vi "Add Children.vi"(8 "Error In":errorcluster, 10 "Parent Index":i32, 11 "DFS Data In":T1) -> (0 "Error Out":errorcluster, 3 "DFS Data Out":T1)   [LabVIEW 2022 SP3]
doc: "<add documentation here>"
uses:
  DFS Data (cluster).ctl
  DFS Node (cluster).ctl
  DFS Child Node (cluster).ctl
panel:
  # "Development\nControls or indicators that are useful for development or testing, but which are not outputs of the VI."
  # "Input\nInputs to the VI"
  # "Output\nOutputs of the VI"
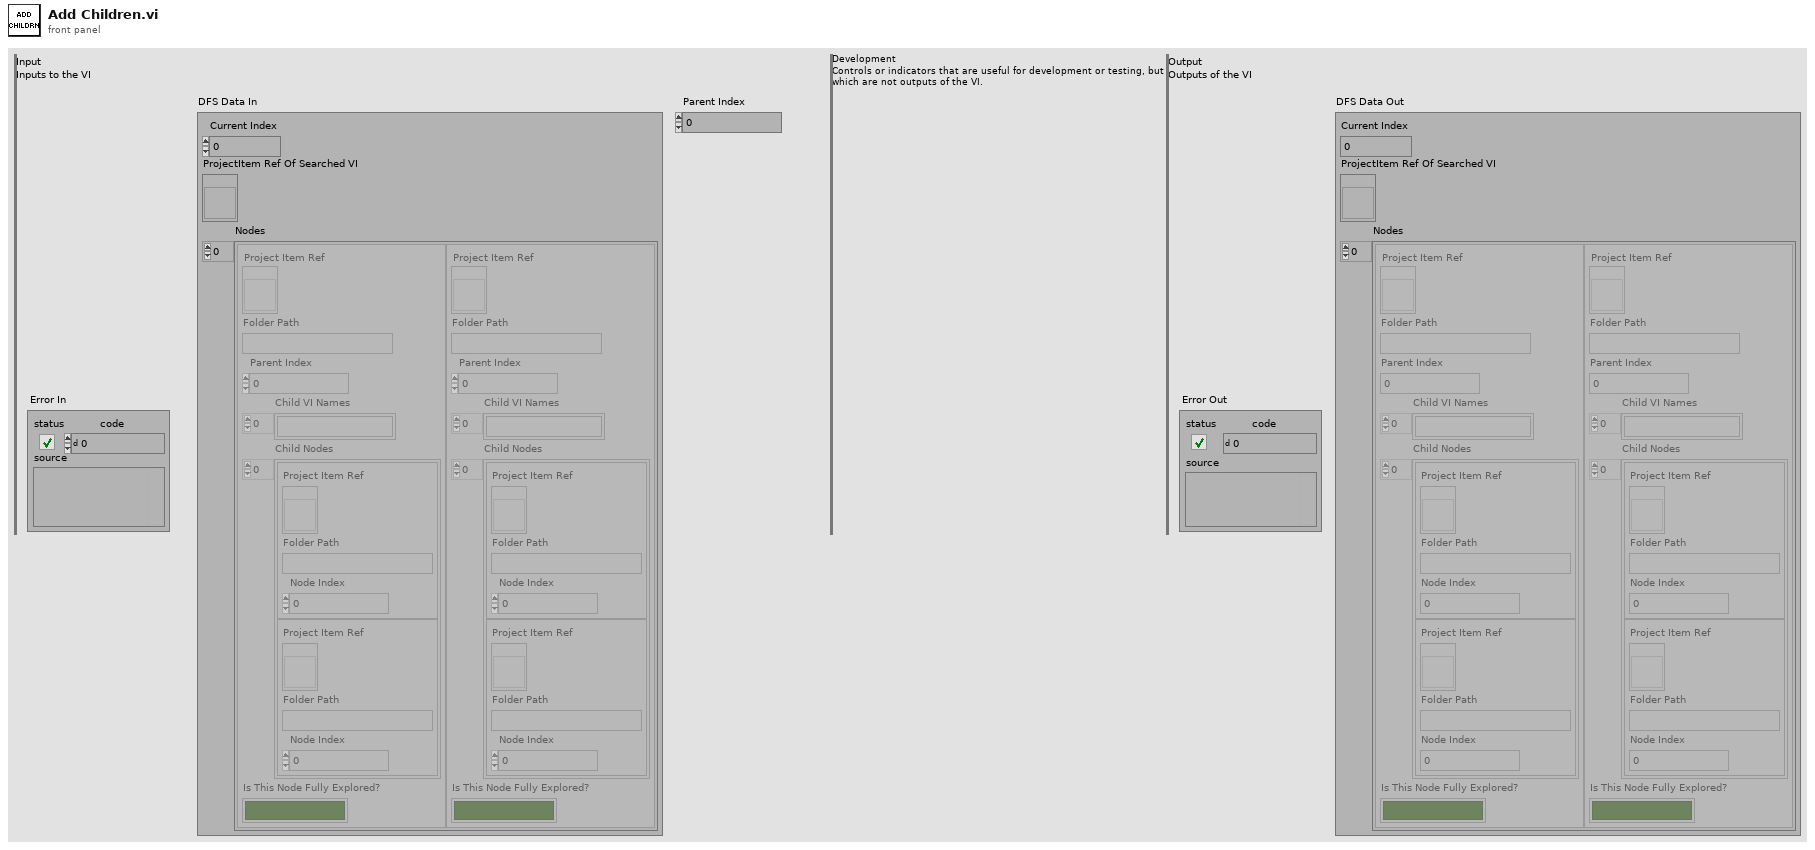
[diagram p1: front panel]
types:
  T1 = typedef "DFS Data (cluster).ctl" = cluster{"Current Index":i32, "ProjectItem Ref Of Searched VI":refnum<vi>, "Nodes":T2[]}
  T2 = typedef "DFS Node (cluster).ctl" = cluster{"Project Item Ref":refnum<vi>, "Folder Path":string, "Parent Index":i32, "Child VI Names":string[], "Child Nodes":T3[], "Is This Node Fully Explored?":bool}
  T3 = typedef "DFS Child Node (cluster).ctl" = cluster{"Project Item Ref":refnum<vi>, "Folder Path":string, "Node Index":i32}
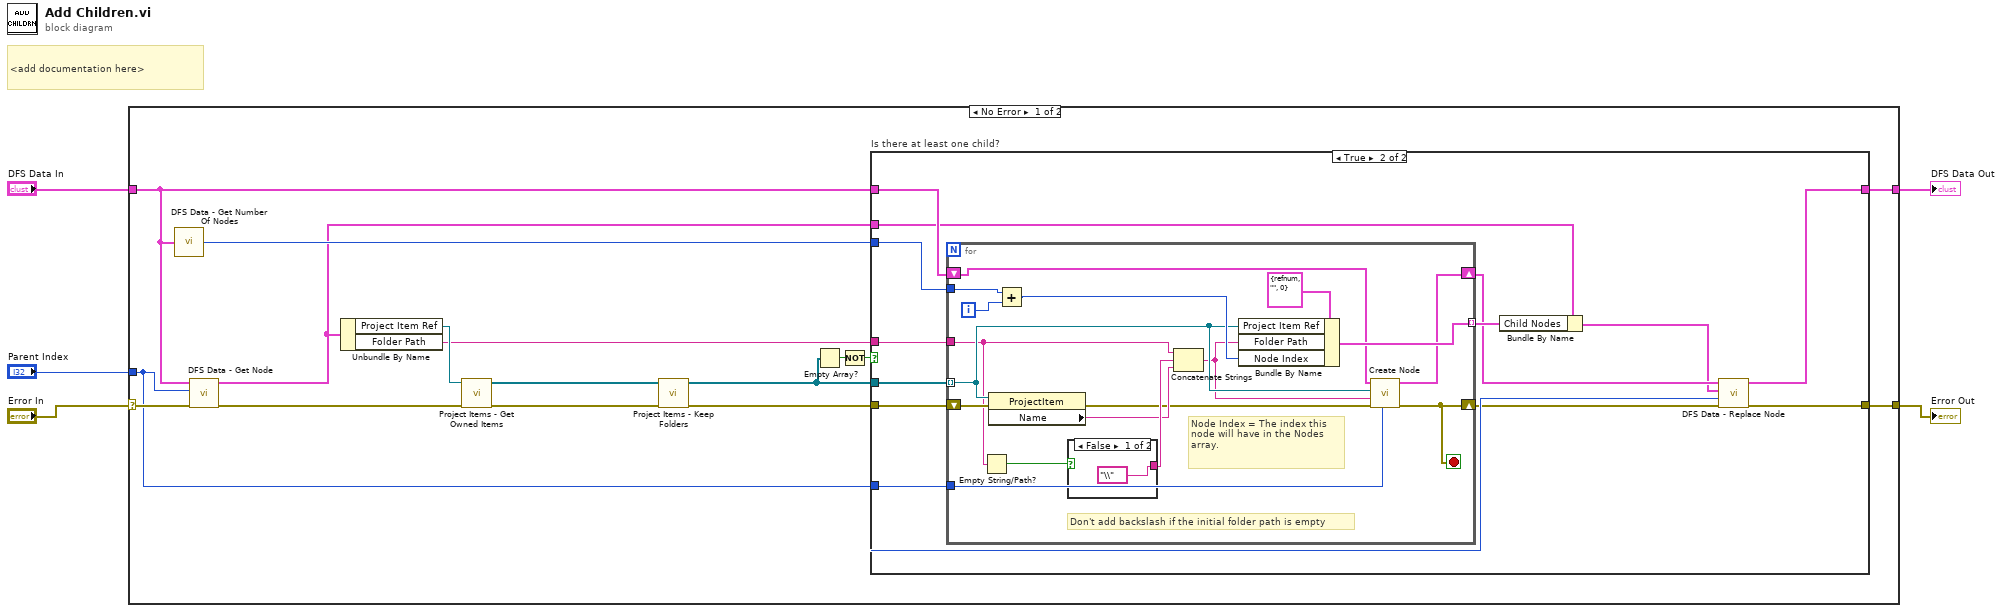
[diagram p0: block diagram]
diagram:
  # "<add documentation here>"
  n1 = case shown="No Error" "Error In" {
    selector: "Error In" -> [w18 w56]
    tunnel: [w9 w56] -> w4
    tunnel: "Parent Index" -> [w10 _]
    tunnel: "DFS Data In" -> [w13 w55]
    tunnel: [w11 w55] -> w1
    frame No Error {
      n2 = call "DFS Data - Get Number Of Nodes.vi"("DFS Data"=w13) -> ("Number Of Nodes"=w14:i32)
      n3 = call "DFS Data - Get Node.vi"("Error In"=w18, "Node Index"=w10, "DFS Data"=w13) -> ("Error Out"=w17:errorcluster, "DFS Node"=w12:T2)  [unwired: 7 in]
      n4 = Unbundle By Name(w12) -> ("Project Item Ref"=w16:refnum<vi>, "Folder Path"=w15:string)
      n5 = call "Project Items - Get Owned Items.vi"("Error In"=w17, "Project Item"=w16) -> ("Error Out"=w21:errorcluster, "Owned Items"=w19:refnum<vi>[])  [unwired: 8 in]
      n6 = call "Project Items - Keep Folders.vi"("Error In"=w21, "Project Items"=w19) -> ("Error Out"=w20:errorcluster, "Project Items (Folders)"=w8:refnum<vi>[])  [unwired: 8 in]
      n7 = Empty Array?(array=w8) -> (empty?=w7:bool)
      n8 = Not(x=w7) -> (.not. x?=w6:bool)
      n9 = case "Is there at least one child?" shown="True" w6 {
        tunnel: w20 -> [w23 w36]
        tunnel: w8 -> [_ w35]
        tunnel: w15 -> [_ w33]
        tunnel: w14 -> [_ w32]
        tunnel: w13 -> [w22 w31]
        tunnel: w12 -> [_ w30]
        tunnel: [w22 w28] -> w11
        tunnel: w10 -> [_ w26]
        tunnel: [w23 w24] -> w9
        frame False {
        }
        frame True {
          n10 = for {
            shift-right: [w44] -> w25
            shift-left: w36 -> [w51]
            tunnel: w35 -> [w41] mode=indexing
            tunnel: [w52] -> w34 mode=indexing
            tunnel: w33 -> [w38]
            tunnel: w32 -> [w48]
            shift-right: [w42] -> w29
            shift-left: w31 -> [w43]
            tunnel: w26 -> [w39]
            i -> [w47]
            stop <- w44 stop-if-true
            # "Don't add backslash if the initial folder path is empty"
            # "Node Index = The index this node will have in the Nodes array."
            n11 = Empty String/Path?(string/path=w38) -> (empty?=w37:bool)
            n12 = property class="ProjectItem"(reference=w41, error in=w51) -> (error out=w45:errorcluster, "Name"=w49:string)  [unwired: 1 out]
            n13 = Add(x=w48, y=w47) -> (x+y=w46:i32)
            n14 = case shown="False" w37 {
              tunnel: ["\\" ("string") _] -> w50
              frame False {
              }
              frame True {
              }
            }
            n15 = Concatenate Strings(w38, w50, w49) -> (w40:string)
            n16 = Bundle By Name(cluster=T3 {"Project Item Ref"=refnum, "Folder Path"="", "Node Index"=0} ("DFS Child Node"), "Project Item Ref"=w41, "Folder Path"=w40, "Node Index"=w46) -> (w52:T3)
            n17 = call "Create Node.vi"("Parent Index"=w39, "Error In"=w45, "Folder Path"=w40, "Project Item"=w41, "DFS Data In"=w43) -> ("Error Out"=w44:errorcluster, "DFS Data Out"=w42:T1)  [unwired: 5 in]
          }
          n18 = Bundle By Name(cluster=w30, "Child Nodes"=w34) -> (w27:T2)
          n19 = call "DFS Data - Replace Node.vi"("Error In"=w25, "Node Index"=w26, "New Node Value"=w27, "DFS Data In"=w29) -> ("Error Out"=w24:errorcluster, "DFS Data Out"=w28:T1)  [unwired: 6 in]
        }
      }
    }
    frame Error {
    }
  }
  "Error Out" <- w4
  "DFS Data Out" <- w1
